vi "Import CSV Files.vi"(8 "error in (no error)":errorcluster, 10 "TopLevel in":T1, 11 "QSM in":string[](array[string])) -> (0 "error out":errorcluster, 2 "TopLevel out":T1, 3 "QSM out":string[](array[string]))   [LabVIEW 2011]
uses:
  Controls/Top Level Control.ctl
  <vilib>/NI/AMC/Message Queue.ctl
  <vilib>/NI/AMC/Message.ctl
  <vilib>/NI/Tools/Keyed Array/KeyedArray.ctl
  Controls/ListBox Test Record.ctl
  Controls/DVR of CSV Tests Data.ctl
  Controls/CSVs Tests Data.ctl
  Controls/Test Column Data.ctl
  Controls/Options DVR.ctl
  Controls/Options.ctl
  <vilib>/NI/Tools/Keyed Array/Tools_KeyedArray.lvlib
  <vilib>/NI/AMC/AMC.lvlib
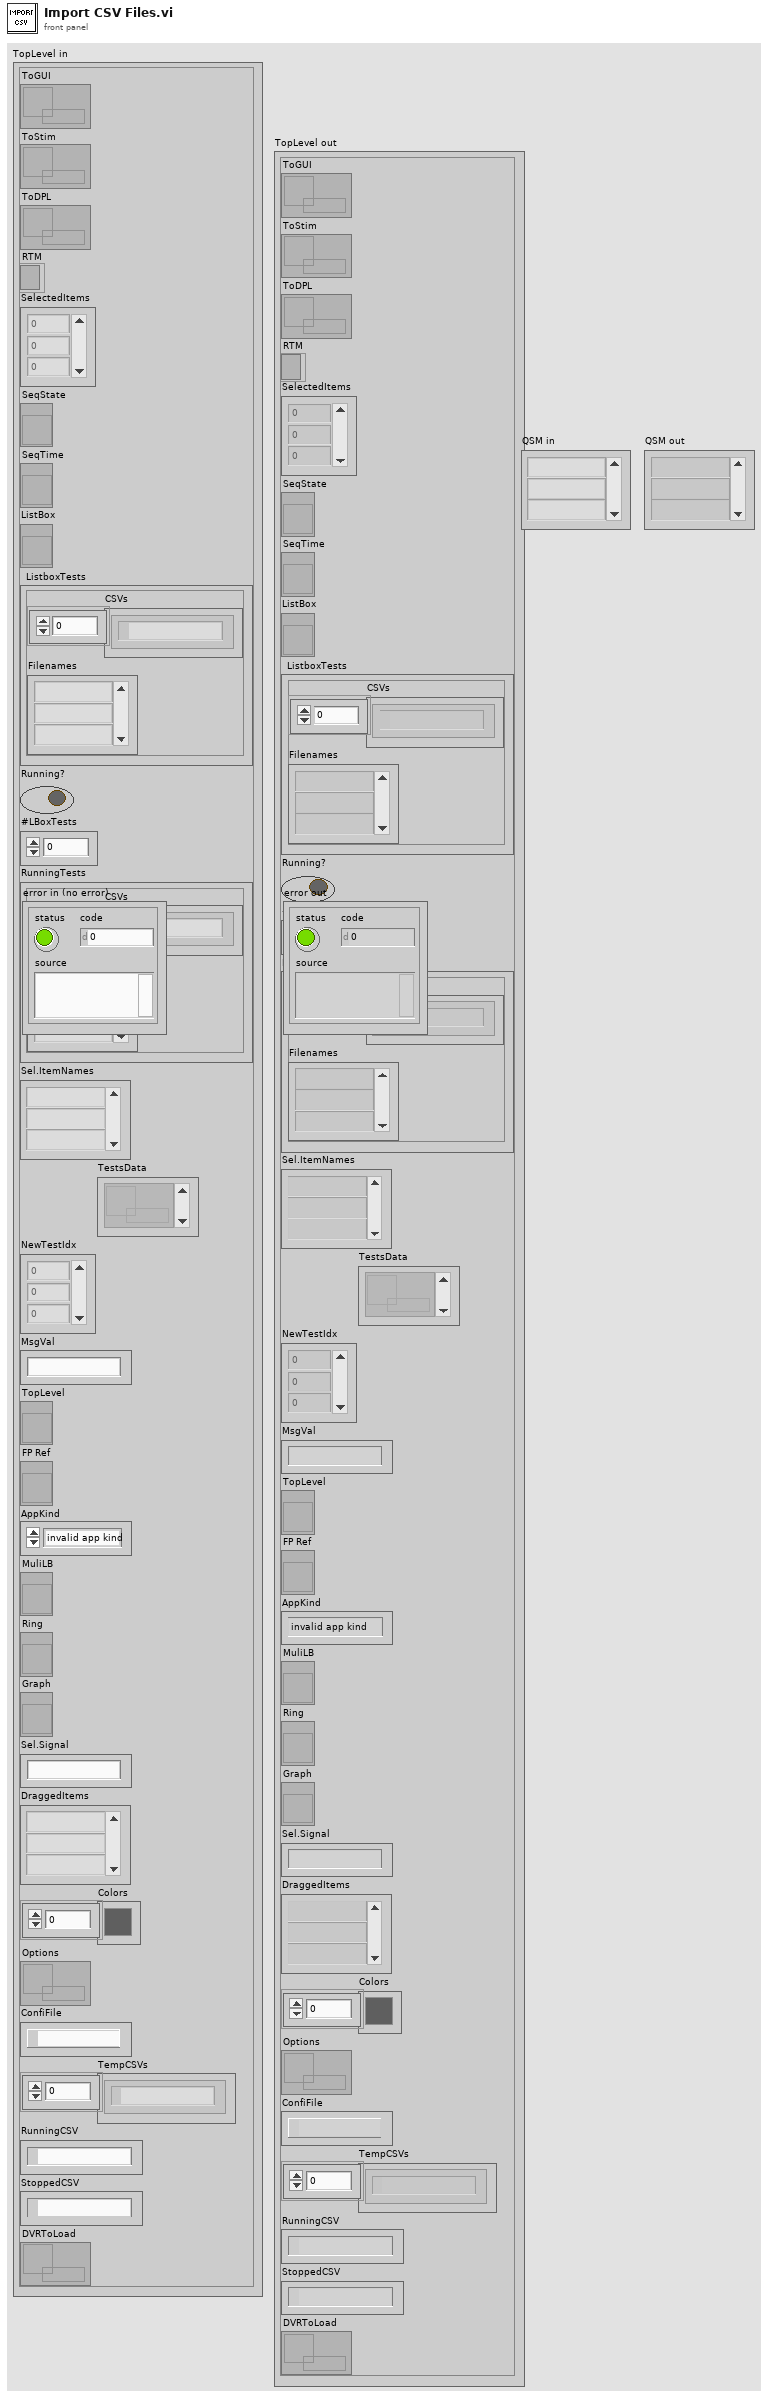
[diagram p1: front panel]
types:
  T1 = typedef "Top Level Control.ctl" = cluster{"ToGUI":T2, "ToStim":T2, "ToDPL":T2, "RTM":refnum<k9>, "SelectedItems":i32[], "SeqState":refnum<vi>, "SeqTime":refnum<vi>, "ListBox":refnum<vi>, "ListboxTests":T3, "Running?":bool, "#LBoxTests":i32, "RunningTests":T3, "Sel.ItemNames":string[], "TestsData":T4[], "NewTestIdx":i32[], "MsgVal":string, "TopLevel":refnum<vi>, "FP Ref":refnum<vi>, "AppKind":enum32{"invalid app kind", "Development System", "Run Time System", "Student Edition", "Embedded LabVIEW", "Evaluation", "Custom"}, "MuliLB":refnum<vi>, "Ring":refnum<vi>, "Graph":refnum<vi>, "Sel.Signal":string, "DraggedItems":string[], "Colors":u32[], "Options":T5, "ConfiFile":path, "TempCSVs":path[], "RunningCSV":path, "StoppedCSV":path, "DVRToLoad":T4}
  T2 = typedef "AMC.lvlib/Message Queue.ctl" = refnum<queue>
  T3 = typedef "ListBox Test Record.ctl" = cluster{"CSVs":path[], "Filenames":string[]}
  T4 = typedef "DVR of CSV Tests Data.ctl" = refnum<data-value>
  T5 = typedef "Options DVR.ctl" = refnum<data-value>
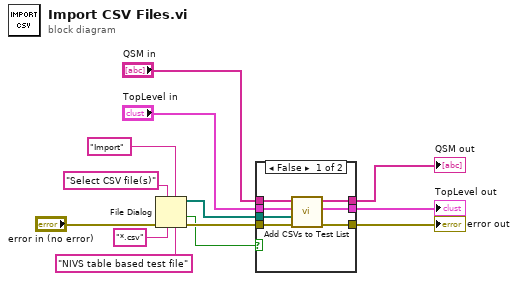
[diagram p0: block diagram]
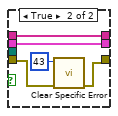
[diagram p2: hidden frame]
diagram:
  n1 = File Dialog(4:"NIVS table based test file" ("pattern label"), 5:"Import" ("button label"), 6:"*.csv" ("pattern (all files)"), 7:"Select CSV file(s)" ("prompt"), 8:"error in (no error)") -> (0:w12:errorcluster, 1:w1:bool, 3:w13:path[])  [unwired: 2 in, 1 out]
  n2 = case shown="False" w1 {
    tunnel: w13 -> [w20 _]
    tunnel: w12 -> [w19 w23]
    tunnel: [w18 w22] -> w11
    tunnel: [w17 w24] -> w5
    tunnel: "QSM in" -> [w16 w24]
    tunnel: [w15 w25] -> w3
    tunnel: "TopLevel in" -> [w14 w25]
    frame False {
      n3 = call "Add CSVs to Test List.vi"("error in (no error)"=w19, "Array"=w20, "TopLevel in in"=w14, "QSM in in"=w16) -> ("error out"=w18:errorcluster, "TopLevel in out"=w15:T1, "QSM in out"=w17:string[])  [unwired: 5 in]
    }
    frame True {
      n4 = call "Clear Specific Error.vi"("error in (no error)"=w23, "code"=43) -> ("error out"=w22:errorcluster)  [unwired: 9 in]
    }
  }
  "TopLevel out" <- w3
  "error out" <- w11
  "QSM out" <- w5
